vi "DiffDrvAccelLimit_New.vi"(8 "MaxAngularAcceleration":dbl, 9 "MaxLinearAcceleration":dbl, 10 "TrackWidth":dbl, 11 "LINEARSYSTEM":T1) -> (3 "outDiffDriveAccelLimit":T3)   [LabVIEW 2019, in "Trajectory_Library.lvlib"]
doc: "Calculate the accelerationlimited differential drive output voltages \nInputs:\n - DiffDriveAccelLimit -- Data cluster\n\nOutputs:\n - Error -- If TRUE, an error occured."
uses:
  DIFF_DRIVE_ACCEL_LIMIT.ctl
  LINEAR_SYSTEM.ctl
  <vilib>/Analysis/Matrix/Datatypes/RealMatrix.ctl
  MatBuilder_Create.vi
  Trajectory_Library.lvlib
  <vilib>/Analysis/Matrix/NI_Matrix.lvlib
panel:
  # "<States,States>"
  # "<States,Inputs>"
  # "<Outputs,States>"
  # "<Outputs,Inputs>"
  # "<States,States>"
  # "<States,Inputs>"
  # "<Outputs,States>"
  # "<Outputs,Inputs>"
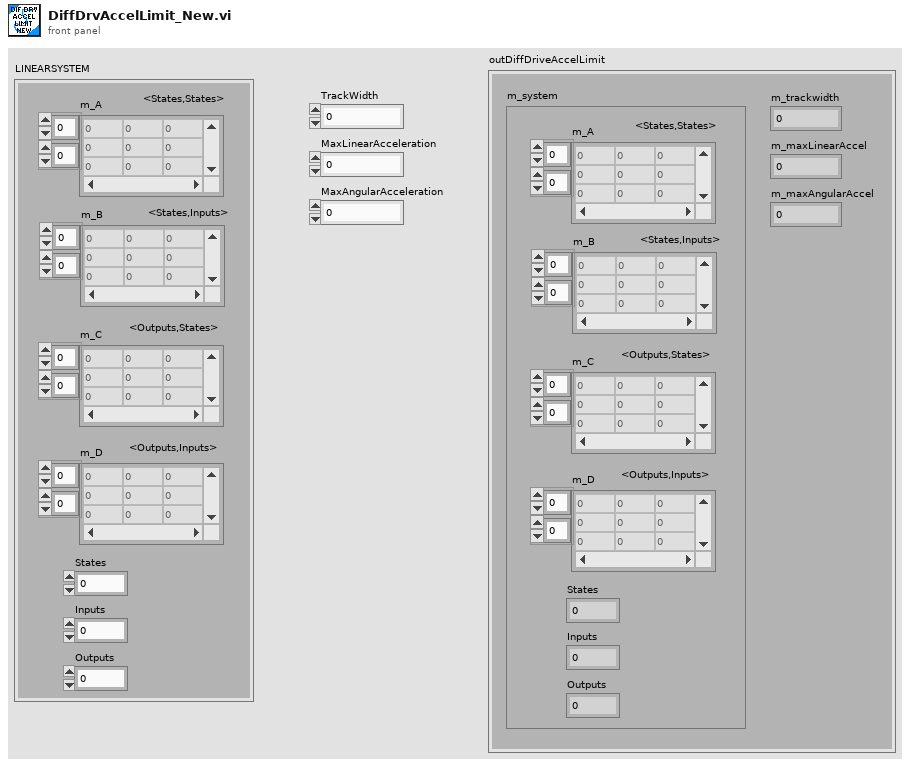
[diagram p1: front panel]
types:
  T1 = typedef "Trajectory_Library.lvlib/LINEAR_SYSTEM.ctl" = cluster{"m_A":T2, "m_B":T2, "m_C":T2, "m_D":T2, "States":i32, "Inputs":i32, "Outputs":i32}
  T2 = typedef "NI_Matrix.lvlib/RealMatrix.ctl" = dbl[][]
  T3 = typedef "Trajectory_Library.lvlib/DIFF_DRIVE_ACCEL_LIMIT.ctl" = cluster{"m_system":T1, "m_trackwidth":dbl, "m_maxLinearAccel":dbl, "m_maxAngularAccel":dbl}
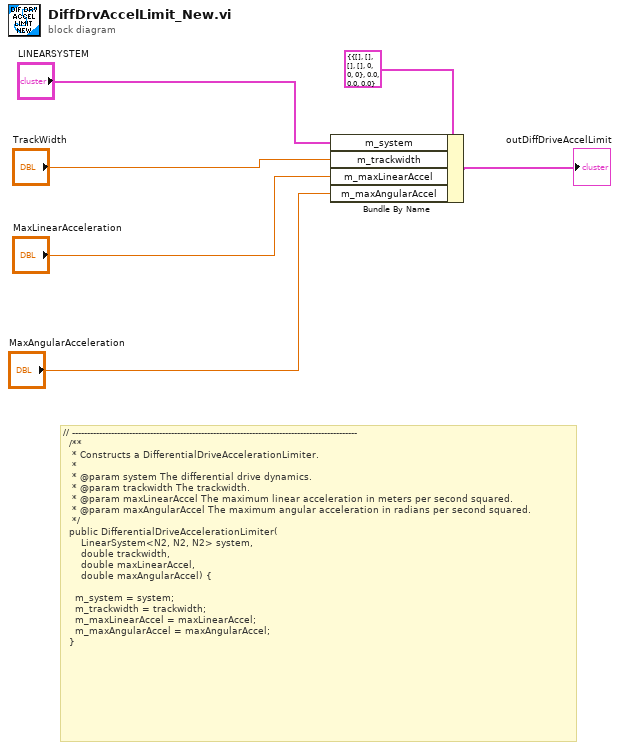
[diagram p0: block diagram]
diagram:
  # "// -----------------------------------------------------------------------------------------------\n  /**\n   * Constructs a DifferentialDriveAccelerationLimiter.\n   *\n   * @param system The differential drive dynamics.\n   * @param trackwidth The trackwidth.\n   * @param maxLinearAccel The maximum linear acceleration in meters per second squared.\n   * @param maxAngularAccel The maximum angular acceleration in radians per second squared.\n   */\n  public DifferentialDriveAccelerationLimiter(\n      LinearSystem<N2, N2, N2> system,\n      double trackwidth,\n      double maxLinearAccel,\n      double maxAngularAccel) {\n\n    m_system = system;\n    m_trackwidth = trackwidth;\n    m_maxLinearAccel = maxLinearAccel;\n    m_maxAngularAccel = maxAngularAccel;\n  }"
  n1 = Bundle By Name(cluster=T3 {"m_system"={"m_A"=[], "m_B"=[], "m_C"=[], "m_D"=[], "States"=0, "Inputs"=0, "Outputs"=0}, "m_trackwidth"=0.0, "m_maxLinearAccel"=0.0, "m_maxAngularAccel"=0.0} ("DIFF_DRIVE_ACCEL_LIMIT"), "m_system"="LINEARSYSTEM", "m_trackwidth"="TrackWidth", "m_maxLinearAccel"="MaxLinearAcceleration", "m_maxAngularAccel"="MaxAngularAcceleration") -> (→"outDiffDriveAccelLimit":T3)
